vi "Parallel Integration Calculation.vi"(6 "Reinit":bool, 7 "i-zone":dbl format="%.2f", 8 "dT":dbl, 9 "PID gains":T1, 10 "Integration Error":dbl, 11 "Curr Error":dbl) -> (2 "Integral Used":bool, 3 "Integral Term":dbl)   [LabVIEW 2020]
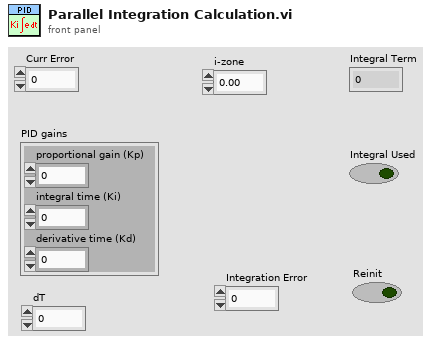
[diagram p1: front panel]
types:
  T1 = cluster{"proportional gain (Kp)":dbl, "integral time (Ki)":dbl, "derivative time (Kd)":dbl}
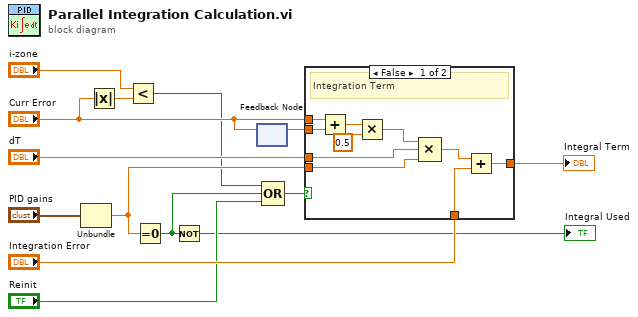
[diagram p0: block diagram]
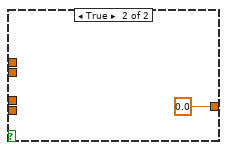
[diagram p2: hidden frame]
diagram:
  n1 = Unbundle("PID gains") -> ("integral time (Ki)"=w9:dbl)  [unwired: 2 out]
  n2 = Absolute Value(x="Curr Error") -> (abs(x)=w3:dbl)
  n3 = Less?(x="i-zone", y=w3) -> (x < y?=w1:bool)
  n4 = Equal To 0?(x=w9) -> (x = 0?=w7:bool)
  n5 = Not(x=w7) -> (.not. x?=→"Integral Used":bool)
  n6 = feedback-in #1("Curr Error") -> ()
  n7 = feedback #1() -> (w10:dbl)  [unwired: 1 in]
  n8 = Compound Arithmetic op=OR(w1, w7, "Reinit") -> (w6:bool)
  n9 = case shown="False" w6 {
    tunnel: w10 -> [w22 _]
    tunnel: "Curr Error" -> [w21 _]
    tunnel: "dT" -> [w19 _]
    tunnel: w9 -> [w18 _]
    tunnel: [w15 0.0] -> w13
    tunnel: "Integration Error" -> [w17 _]
    frame False {
      # "Integration Term"
      n10 = Add(x=w21, y=w22) -> (x+y=w23:dbl)
      n11 = Multiply(x=w23, y=0.5) -> (x*y=w20:dbl)
      n12 = Compound Arithmetic op=MULTIPLY(w20, w19, w18) -> (w16:dbl)
      n13 = Add(x=w16, y=w17) -> (x+y=w15:dbl)
    }
    frame True {
    }
  }
  "Integral Term" <- w13
